vi "tm_opencamera.vi"(7 "Force Open":bool, 8 "error in (no error)":errorcluster {"code" format="%.0x"}, 11 "Camera Index":u32) -> (0 "error out":errorcluster {"code" format="%.0x"}, 2 "Camera Details":T1, 3 "Handle out":u32)   [LabVIEW 2011]
uses:
  tmcamcon.dll
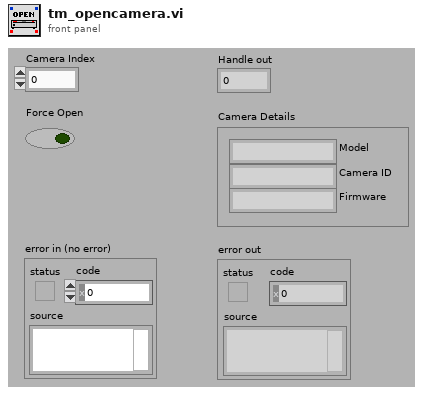
[diagram p1: front panel]
types:
  T1 = cluster{"Model":string, "Camera ID":string, "Firmware":string}
  T2 = cluster{"string":string, "string":string, "string":string}
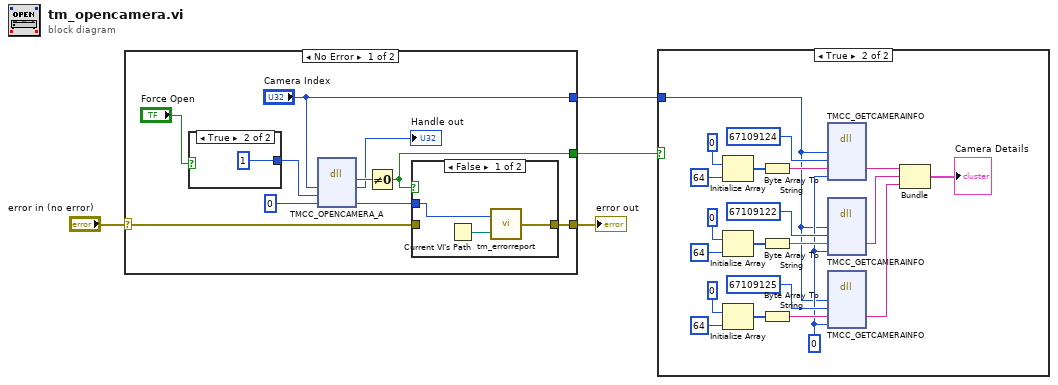
[diagram p0: block diagram]
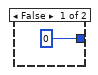
[diagram p4: hidden frame]
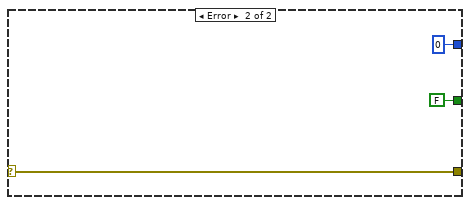
[diagram p5: hidden frame]
diagram:
  n1 = case shown="No Error" "error in (no error)" {
    selector: "error in (no error)" -> [w9 w23]
    tunnel: [w8 w23] -> w3
    tunnel: [w6 FALSE] -> w2
    tunnel: ["Camera Index" u32 0 ("Camera Index")] -> w1
    frame No Error {
      n2 = case shown="True" "Force Open" {
        tunnel: [0 1] -> w10
        frame False {
        }
        frame True {
        }
      }
      n3 = dll-call lib="tmcamcon.dll" fn="TMCC_OPENCAMERA_A"("i"="Camera Index", "force"=w10, "Erval"=0) -> ("return type"=w14:u32, "i"=→"Handle out":u32, "Erval"=w7:i32)  [unwired: 4 in, 2 out]
      n4 = Not Equal To 0?(x=w14) -> (x != 0?=w6:bool)
      n5 = case shown="False" w6 {
        tunnel: w9 -> [_ w18]
        tunnel: [w16 w18] -> w8
        tunnel: w7 -> [w15 _]
        frame False {
          n6 = Current VI's Path() -> (path=w17:path)
          n7 = call <userlib>:"tm_errorreport.vi"("Source"=w17, "Error"=w15) -> ("error out"=w16:errorcluster)
        }
        frame True {
        }
      }
    }
    frame Error {
    }
  }
  "error out" <- w3
  n8 = case shown="True" w2 {
    tunnel: w1 -> [_ w25]
    frame False {
    }
    frame True {
      w26 = 0 ("Erval")
      n9 = Initialize Array(u8 0, 64) -> (w44:u8[])
      n10 = Initialize Array(u8 0, 64) -> (w39:u8[])
      n11 = Initialize Array(u8 0, 64) -> (w34:u8[])
      n12 = Byte Array To String(unsigned byte array=w44) -> (string=w40:string)
      n13 = Byte Array To String(unsigned byte array=w39) -> (string=w35:string)
      n14 = Byte Array To String(unsigned byte array=w34) -> (string=w30:string)
      n15 = dll-call lib="tmcamcon.dll" fn="TMCC_GETCAMERAINFO"("index"=w25, "ID"=u32 67109124, "string"=w40, "Erval"=w26) -> ("string"=w29:string)  [unwired: 7 in, 2 out]
      n16 = dll-call lib="tmcamcon.dll" fn="TMCC_GETCAMERAINFO"("index"=w25, "ID"=u32 67109122, "string"=w35, "Erval"=w26) -> ("string"=w28:string)  [unwired: 7 in, 2 out]
      n17 = dll-call lib="tmcamcon.dll" fn="TMCC_GETCAMERAINFO"("index"=w25, "ID"=u32 67109125, "string"=w30, "Erval"=w26) -> ("string"=w27:string)  [unwired: 7 in, 2 out]
      n18 = Bundle("string"=w29, "string"=w28, "string"=w27) -> (→"Camera Details":T2)  [unwired: 1 in]
    }
  }
